vi "Launch All.vi"(8 "error in (no error)":errorcluster, 11 "Thread Manager in":refnum<class "Thread Manager.lvclass">) -> (0 "error out":errorcluster, 3 "Thread Manager out":refnum<class "Thread Manager.lvclass">)   [LabVIEW 2021, in "DSF Core.lvlib" / "Thread Manager.lvclass"]
uses:
  Thread Manager.lvclass
  Thread Manager.lvclass/Thread Manager.ctl
  Thread/Thread.lvclass/Thread.ctl
  Thread/Top.vi
  Thread/Thread.lvclass
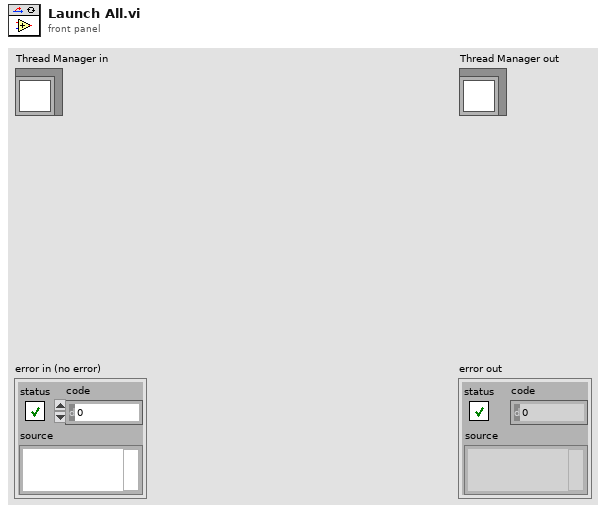
[diagram p1: front panel]
types:
  T1 = typedef "DSF Core.lvlib/Thread.lvclass/Thread Options.ctl" = cluster{"Show FP On Call":bool, "Close FP After Call":bool, "Allow Debugging":bool}
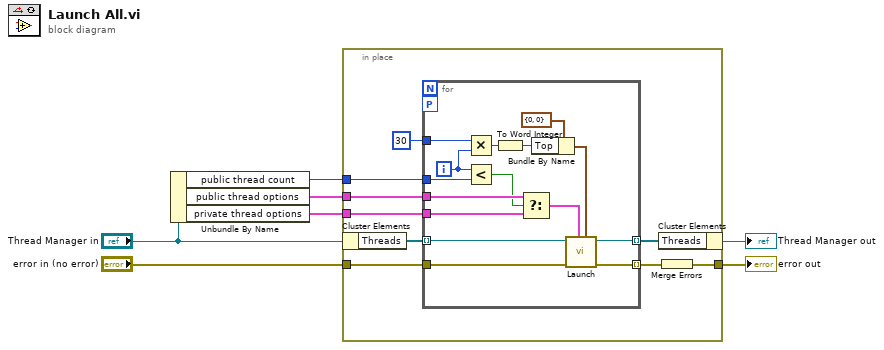
[diagram p0: block diagram]
diagram:
  n1 = Unbundle By Name("Thread Manager in") -> ("public thread count"=w3:i32, "public thread options"=w4:T1, "private thread options"=w5:T1)
  n2 = in-place {
    in-place-border: "error in (no error)" -> [w16]
    in-place-border: [w8] -> w1
    in-place-border: w5 -> [w12]
    in-place-border: w4 -> [w11]
    in-place-border: w3 -> [w10]
    n3 = in-place-cluster #1("Thread Manager in") -> ("Threads"=w14:refnum<class "Thread.lvclass">[])
    n4 = for {
      tunnel: w14 -> [w29] mode=indexing
      tunnel: [w28] -> w13 mode=indexing
      tunnel: w12 -> [w25]
      tunnel: w11 -> [w27]
      tunnel: w10 -> [w23]
      workers-P: _ -> [_]
      tunnel: 30 ("x") -> [w21]
      tunnel: w16 -> [w31]
      tunnel: [w30] -> w15 mode=indexing
      i -> [w22]
      n5 = Multiply(x=w21, y=w22) -> (x*y=w20:i32)
      n6 = Less?(x=w22, y=w23) -> (x < y?=w24:bool)
      n7 = To Word Integer(number=w20) -> (16bit integer=w17:i16)
      n8 = Select(t=w27, s=w24, f=w25) -> (s? t:f=w26:T1)
      n9 = Bundle By Name(cluster=cluster{"Left":i16, "Top":i16} {"Left"=0, "Top"=0} ("window position"), "Top"=w17) -> (w18:cluster{"Left":i16, "Top":i16})
      n10 = call "Launch.vi"("window position"=w18, "options"=w26, "error in (no error)"=w31, "Thread in"=w29) -> ("error out"=w30:errorcluster, "Thread out"=w28:refnum<class "Thread.lvclass">)  [unwired: 6 in]
    }
    n11 = in-place-cluster #1("Threads"=w13) -> (→"Thread Manager out":refnum<class "Thread Manager.lvclass">)
    n12 = Merge Errors(w15) -> (w8:errorcluster)
  }
  "error out" <- w1
